vi "Create MetaData Channel - Array - Type Cast.vi"(8 "error in (no error)":errorcluster, 9 "settings":T2, 10 "channel name":string, 11 "command refnum in":T1=18446744073709551615 format="%.0x") -> (0 "error out":errorcluster, 1 "channel refnums":T1[](array[typedef]) format="%.0x", 2 "array refnum":T1=18446744073709551615 format="%.0x", 3 "command refnum out":T1=18446744073709551615 format="%.0x")   [LabVIEW 2018, in "Instrument Addon Scripting API.lvlib"]
doc: "Creates a new metadata channel array under the specified command."
uses:
  Instrument Addon Scripting API.lvlib
  <vilib>/NI Veristand/Custom Device API/Custom Device Item Ref.ctl
  TypeDefs/Array Type Cast Settings.ctl
  TypeDefs/Array Element.ctl
  Addon/Addon Shared/Types/Type Cast Type.ctl
  Addon/Addon Shared/Types/Endian.ctl
  Addon/Addon Shared/Types/MetaData Parameters.ctl
  Addon/Addon Shared/Types/Protocol Data Type.ctl
  Addon/Addon Shared/Types/Metadata Channel Type.ctl
  Addon/Addon Shared/Instrument Addon Shared.lvlib
  <vilib>/NI Veristand/Custom Device API/Custom Device API.lvlib
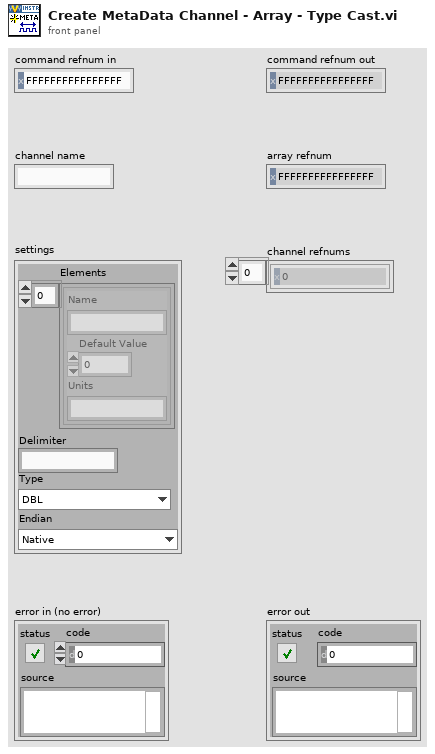
[diagram p1: front panel]
types:
  T1 = typedef "Custom Device API.lvlib/Custom Device Item Ref.ctl" = u64
  T2 = typedef "Instrument Addon Scripting API.lvlib/Array Type Cast Settings.ctl" = cluster{"Elements":T3[], "Delimiter":string, "Type":T4, "Endian":T5}
  T3 = typedef "Instrument Addon Scripting API.lvlib/Array Element.ctl" = cluster{"Name":string, "Default Value":dbl, "Units":string}
  T4 = typedef "Instrument Addon Shared.lvlib/Type Cast Type.ctl" = enum16{"DBL", "SGL", "U64", "U32", "U16", "U8", "I64", "I32", "I16", "I8"}
  T5 = typedef "Instrument Addon Shared.lvlib/Endian.ctl" = enum16{"Native", "Little", "Big"}
  T6 = typedef "Instrument Addon Shared.lvlib/Metadata Channel Type.ctl" = enum16{"Enumerated List", "Format", "Type Cast"}
  T7 = typedef "Instrument Addon Shared.lvlib/Protocol Data Type.ctl" = enum16{"Single Channel", "Array"}
  T8 = typedef "Instrument Addon Shared.lvlib/MetaData Parameters.ctl" = cluster{"Data Type":T7, "Channel Type":T6, "List":string[], "Format String":string, "Type":T4, "Delimiter":string, "Endian":T5}
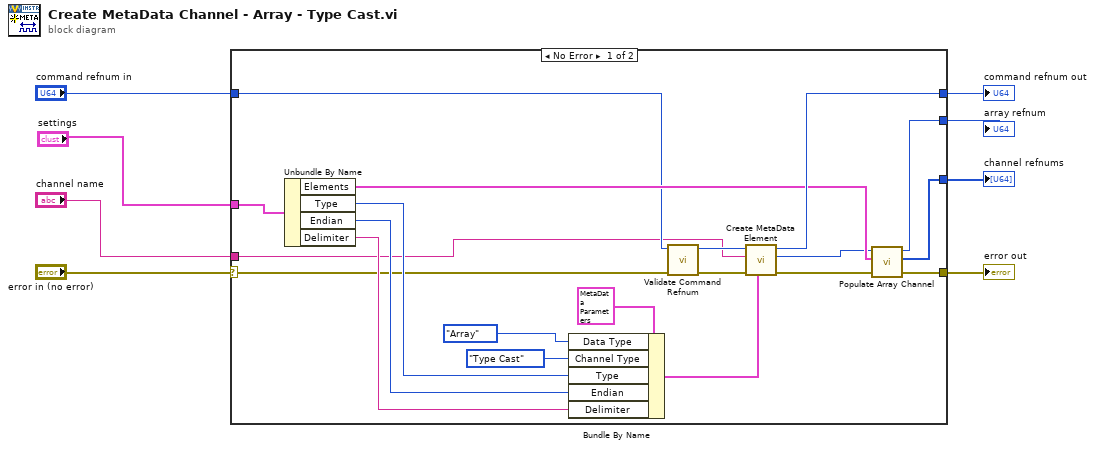
[diagram p0: block diagram]
diagram:
  n1 = case shown="No Error" "error in (no error)" {
    selector: "error in (no error)" -> [w12 w29]
    tunnel: "command refnum in" -> [w10 w30]
    tunnel: [w24 w30] -> w7
    tunnel: "channel name" -> [w9 _]
    tunnel: "settings" -> [w23 _]
    tunnel: [w21 w29] -> w5
    tunnel: [w15 _] -> w2
    tunnel: [w14 _] -> w1
    frame No Error {
      n2 = Unbundle By Name(w23) -> ("Elements"=w17:T3[], "Type"=w20:T4, "Endian"=w19:T5, "Delimiter"=w18:string)
      n3 = Bundle By Name(cluster=T8 {"Data Type"=enum."Single Channel", "Channel Type"=enum."Format", "List"=[], "Format String"="%.3g", "Type"=enum."SGL", "Delimiter"="", "Endian"=enum."Native"} ("MetaData Parameters"), "Data Type"=Protocol_Data_Type."Array", "Channel Type"=Metadata_Channel_Type."Type Cast", "Type"=w20, "Endian"=w19, "Delimiter"=w18) -> (w25:T8)
      n4 = call "Validate Command Refnum.vi"("error in (no error)"=w12, "command refnum in"=w10) -> ("error out"=w13:errorcluster, "command refnum out"=w11:T1)  [unwired: 8 in]
      n5 = call "Create MetaData Element.vi"("MetaData Parameters"=w25, "error in (no error)"=w13, "Name"=w9, "Refnum In"=w11) -> ("error out"=w22:errorcluster, "Channel Refnum"=w16:T1, "Refnum Out"=w24:T1)  [unwired: 5 in]
      n6 = call "Populate Array Channel.vi"("error in (no error)"=w22, "Elements"=w17, "Array Refnum In"=w16) -> ("error out"=w21:errorcluster, "Channel Refnums"=w14:T1[], "Array Refnum Out"=w15:T1)  [unwired: 6 in]
    }
    frame Error {
    }
  }
  "command refnum out" <- w7
  "error out" <- w5
  "array refnum" <- w2
  "channel refnums" <- w1
